vi "Write Registry Cache Array Reference.vi"(8 "error in (no error)":errorcluster, 10 "Registry Cache Array Reference":refnum<data-value>, 11 "navX Registry Cache in":refnum<class "navX Registry Cache.lvclass">) -> (0 "error out":errorcluster, 3 "navX Registry Cache out":refnum<class "navX Registry Cache.lvclass">)   [LabVIEW 2015, in "navX Library v3.lvlib" / "navX Registry Cache.lvclass"]
uses:
  navX Registry Cache.lvclass
  navX Registry Cache.lvclass/navX Registry Cache.ctl
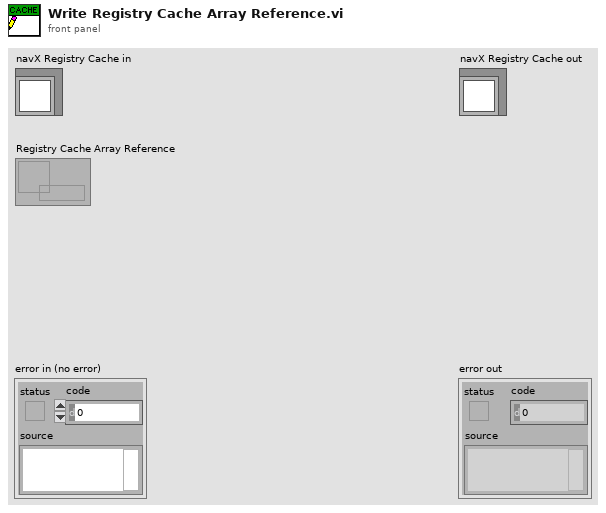
[diagram p1: front panel]
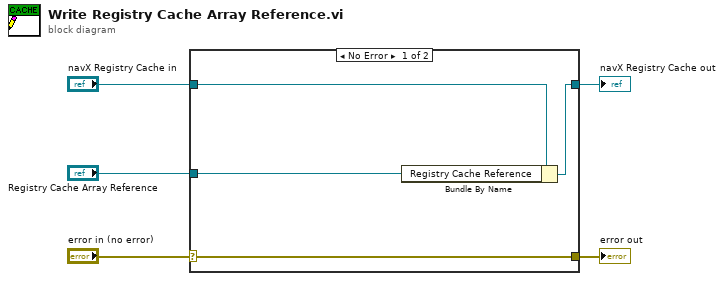
[diagram p0: block diagram]
diagram:
  n1 = case shown="No Error" "error in (no error)" {
    selector: "error in (no error)" -> [w9 w10]
    tunnel: [w9 w10] -> w4
    tunnel: [w7 w11] -> w2
    tunnel: "navX Registry Cache in" -> [w8 w11]
    tunnel: "Registry Cache Array Reference" -> [w6 _]
    frame No Error {
      n2 = Bundle By Name(cluster=w8, "Registry Cache Reference"=w6) -> (w7:refnum<class "navX Registry Cache.lvclass">)
    }
    frame Error {
    }
  }
  "error out" <- w4
  "navX Registry Cache out" <- w2
